vi "Register Indicators.vi"(8 "error in (no error)":errorcluster, 11 "PluginGUI in":refnum<class "PluginGUI.lvclass">) -> (0 "error out":errorcluster, 3 "PluginGUI out":refnum<class "PluginGUI.lvclass">)   [LabVIEW 2020, in "VolatusGUI.lvlib" / "PluginGUI.lvclass"]
uses:
  PluginGUI.lvclass
  C:/dev/lv20CE/relink/lv-volatus/Volatus/Module/Module.lvclass
  Volatus/Module/Module.lvclass/Module.ctl
  PluginGUI.lvclass/PluginGUI.ctl
  Volatus/Module/Module.lvclass
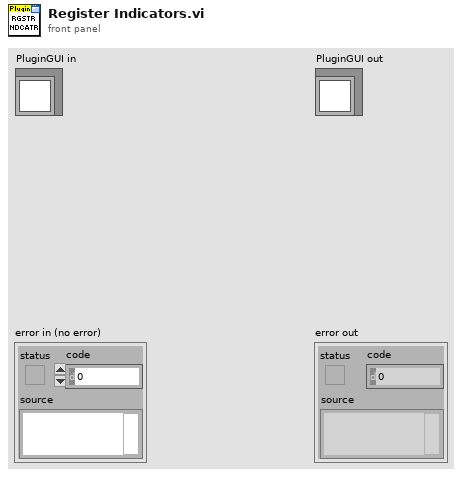
[diagram p1: front panel]
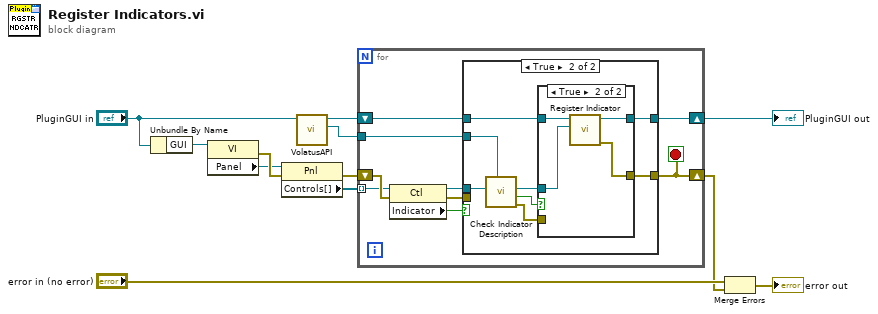
[diagram p0: block diagram]
diagram:
  n1 = Unbundle By Name("PluginGUI in") -> ("GUI"=w10:refnum<vi>)
  n2 = property class="VI"(reference=w10) -> (error out=w12:errorcluster, "Panel"=w9:refnum<vi>)  [unwired: 1 in, 1 out]
  n3 = property class="Pnl"(reference=w9, error in=w12) -> (error out=w8:errorcluster, "Controls[]"=w7:refnum<vi>[])  [unwired: 1 out]
  n4 = call "VolatusAPI.vi"("Module in"="PluginGUI in") -> ("VolatusAPI"=w1:refnum<class "VolatusAPI.lvclass">, "Module out"=w2:refnum<class "PluginGUI.lvclass">)  [unwired: 9 in]
  n5 = for {
    shift-right: [w14] -> w3
    shift-left: w8 -> [w21]
    tunnel: w7 -> [w20] mode=indexing
    shift-right: [w16] -> w5
    shift-left: w2 -> [w17]
    tunnel: w1 -> [w13]
    stop <- w14 stop-if-true
    n6 = property class="Ctl"(reference=w20, error in=w21) -> (reference out=w19:refnum<vi>, error out=w15:errorcluster, "Indicator"=w18:bool)
    n7 = case shown="True" w18 {
      tunnel: w19 -> [_ w31]
      tunnel: w17 -> [w23 w28]
      tunnel: [w23 w25] -> w16
      tunnel: w15 -> [w22 _]
      tunnel: [w22 w26] -> w14
      tunnel: w13 -> [_ w24]
      frame False {
      }
      frame True {
        n8 = call "Check Indicator Description.vi"("VolatusAPI"=w24, "Ref"=w31) -> ("error out"=w27:errorcluster, "Register"=w30:bool, "Indicator"=w29:refnum<class "Indicator.lvclass">)  [unwired: 7 in]
        n9 = case shown="True" w30 {
          tunnel: w29 -> [_ w35]
          tunnel: w28 -> [w32 w37]
          tunnel: w27 -> [w33 _]
          tunnel: [w33 w34] -> w26
          tunnel: [w32 w36] -> w25
          frame False {
          }
          frame True {
            n10 = call "Register Indicator.vi"("VolatusGUI:Indicator"=w35, "PluginGUI in"=w37) -> ("error out"=w34:errorcluster, "PluginGUI out"=w36:refnum<class "PluginGUI.lvclass">)  [unwired: 8 in]
          }
        }
      }
    }
  }
  "PluginGUI out" <- w5
  n11 = Merge Errors("error in (no error)", w3) -> (→"error out":errorcluster)
